vi "test_data_structure.vi"() -> ()   [LabVIEW 2016]
panel:
  out "string 3":string
  out "string 2":string
  out "subarray":u8[](array[numeric])
  out "element":u8
  out "string":string
  out "unsigned 8bit integer":u8[](array[numeric])
  out "double precision float":dbl[](array[numeric])
  out "*(type *) &x":u8[](array[numeric])
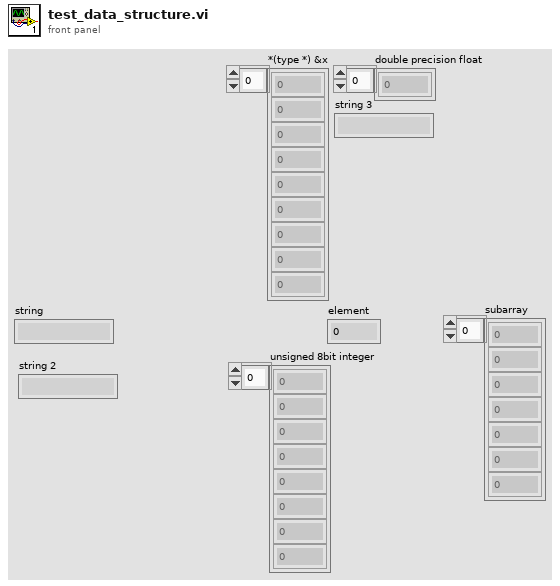
[diagram p1: front panel]
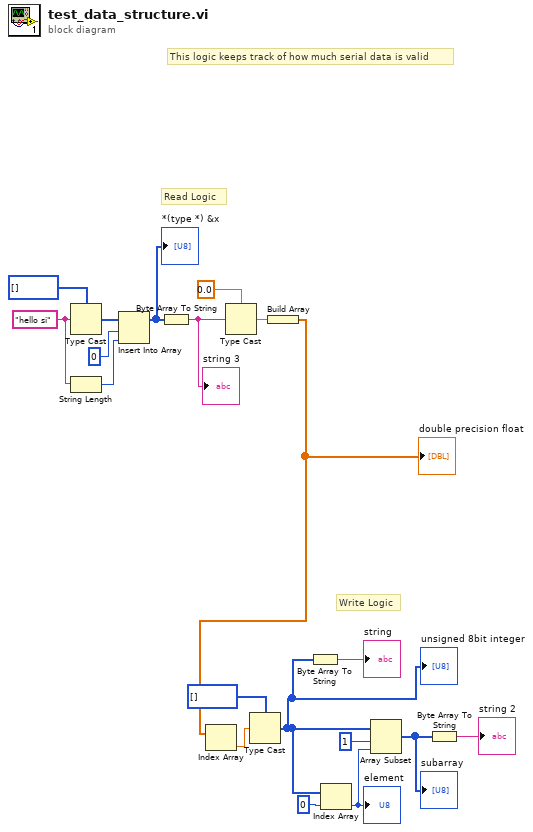
[diagram p0: block diagram]
diagram:
  w16 = "hello si"
  # "Write Logic"
  # "This logic keeps track of how much serial data is valid"
  # "Read Logic"
  n1 = Type Cast(type=u8[] [], x=w16) -> (*(type *) &x=w17:u8[])
  n2 = String Length(string=w16) -> (length=w15:i32)
  n3 = Insert Into Array(array=w17, index=0, new element=w15) -> (w14:u8[])
  "*(type *) &x" <- w14
  n4 = Byte Array To String(unsigned byte array=w14) -> (string=w13:string)
  "string 3" <- w13
  n5 = Type Cast(type=0.0, x=w13) -> (*(type *) &x=w11:dbl)
  n6 = Build Array(w11) -> (w10:dbl[])
  "double precision float" <- w10
  n7 = Index Array(array=w10) -> (element=w9:dbl)  [unwired: 1 in]
  n8 = Type Cast(type=u8[] [], x=w9) -> (*(type *) &x=w1:u8[])
  "unsigned 8bit integer" <- w1
  n9 = Byte Array To String(unsigned byte array=w1) -> (string=→"string":string)
  n10 = Index Array(array=w1, index=0) -> (element=w5:u8)
  "element" <- w5
  n11 = Array Subset(array=w1, index=1, length=w5) -> (w3:u8[])
  "subarray" <- w3
  n12 = Byte Array To String(unsigned byte array=w3) -> (string=→"string 2":string)
